vi "LVClass_Image data equalize AB.vi"(0 "Image A in":refnum<class "Image.lvclass">, 5 "Image B":refnum<class "Image.lvclass">, 11 "error in (no error)":errorcluster) -> (4 "Image A out":refnum<class "Image.lvclass">, 6 "Image B (dup)":refnum<class "Image.lvclass">, 15 "error out":errorcluster)   [LabVIEW 2020, in "Image.lvclass"]
doc: "Assignment : copy ImageB content to ImageA. Images must have the same size,\nchannels count and bits depth.\n\n--------------------------------------------------------------------------------\n\n<B>ImageAIn </B> : Pointer to destination Image object.\n<B>ImageAOut </B> : Pointer to destination Image object.\n<B>ImageB </B> : Pointer to source image object.\n<B>ErrorIn </B> : Error\n<B>ErrorOut </B> : Error\n\n--------------------------------------------------------------------------------"
uses:
  Image.lvclass
  Image.lvclass/Image.ctl
  LVClass_Image read Image Compat ptr.vi
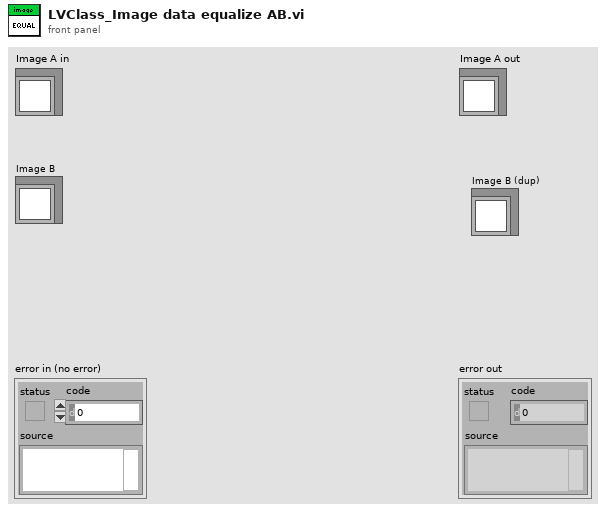
[diagram p1: front panel]
types:
  T1 = typedef "ClassID.ctl" = i64
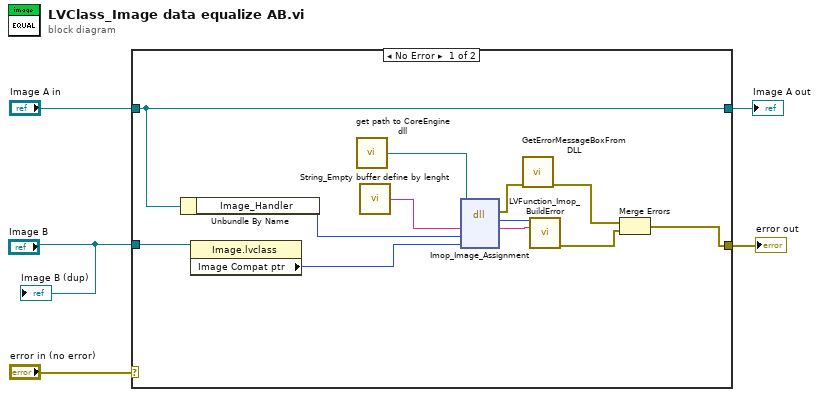
[diagram p0: block diagram]
diagram:
  n1 = case shown="No Error" "error in (no error)" {
    selector: "error in (no error)" -> [_ w19]
    tunnel: [w6 w19] -> w4
    tunnel: [w10 w18] -> w2
    tunnel: "Image A in" -> [w10 w18]
    tunnel: "Image B" -> [w14 _]
    frame No Error {
      n2 = Unbundle By Name(w10) -> ("Image_Handler"=w9:T1)
      n3 = property class="Image.lvclass"(reference=w14) -> ("Image Compat ptr"=w13:T1)  [unwired: 1 in, 2 out]
      n4 = call "get path to CoreEngine dll.vi"() -> ("path to wavekit library"=w12:path)  [unwired: 14 in, 1 out]
      n5 = call "String_Empty buffer define by lenght.vi"() -> ("Empty buffer"=w17:string)  [unwired: 1 in]
      n6 = dll-call lib="D:/soft/HASO_v3/SVN_trunk/ImOpCoreEngine4_LV2011/DLLs/c_interface_vc100.dll" fn="Imop_Image_Assignment"(path in=w12, "message"=w17, "Image 1"=w9, "Image 2"=w13) -> (error out=w11:errorcluster, "return type"=w16:i32, "message"=w15:string)  [unwired: 4 in, 1 out]
      n7 = call "GetErrorMessageBoxFromDLL.vi"("error IN"=w11) -> ("error OUT"=w8:errorcluster)  [unwired: 10 in]
      n8 = call "LVFunction_Imop_BuildError.vi"("code"=w16, "String to Prepend to source (\"\")"=w15) -> ("error out"=w7:errorcluster)  [unwired: 13 in]
      n9 = Merge Errors(w8, w7) -> (w6:errorcluster)
    }
    frame Error {
    }
  }
  "error out" <- w4
  "Image A out" <- w2
  "Image B (dup)" <- "Image B"
